vi "Parse NMEA.vi"(8 "error in (no error)":errorcluster, 11 "NMEA Line":string) -> (0 "error out":errorcluster, 3 "NMEA Message out":refnum<class "NMEA Message.lvclass">)   [LabVIEW 2020, in "nmea.lvlib" / "NMEA Message.lvclass"]
uses:
  NMEA Message.lvclass
  NMEA Message.lvclass/NMEA Message.ctl
  <vilib>/Utility/error.llb/Error Cluster From Error Code.vi
  <vilib>/ErrorRing/Error Ring.xnode
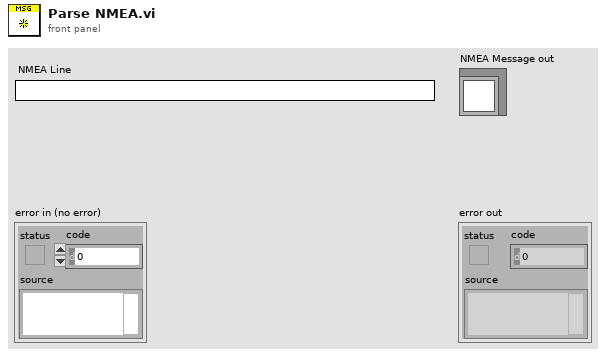
[diagram p1: front panel]
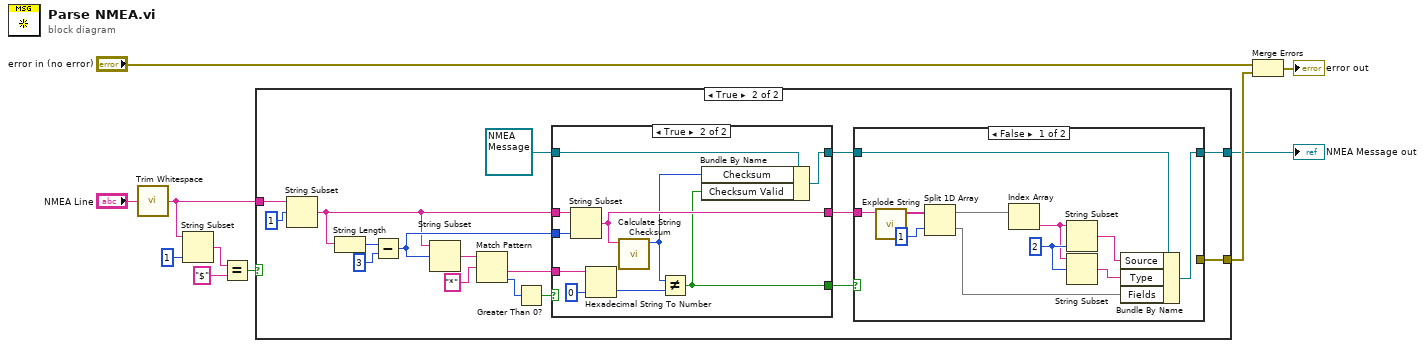
[diagram p0: block diagram]
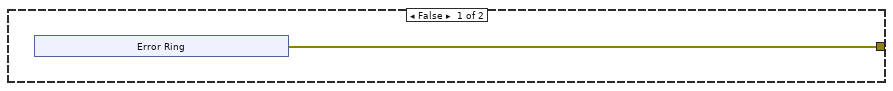
[diagram p2: hidden frame]
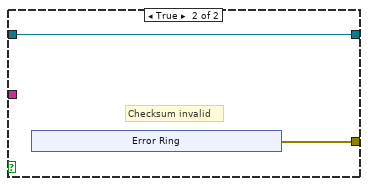
[diagram p4: hidden frame]
diagram:
  n1 = call <vilib>:"Trim Whitespace.vi"("string"="NMEA Line") -> ("trimmed string"=w4:string)  [unwired: 1 in]
  n2 = String Subset(string=w4, length (rest)=1 ("length (rest)")) -> (substring=w8:string)  [unwired: 1 in]
  n3 = Equal?(x=w8, y="$") -> (x = y?=w6:bool)
  n4 = case shown="True" w6 {
    tunnel: w4 -> [_ w15]
    tunnel: [_ w17] -> w1
    tunnel: [w11 w16] -> w2
    frame False {
      n5 = xnode "Error Ring"() -> ("error out"=w11:errorcluster)
    }
    frame True {
      n6 = String Subset(string=w15, offset (0)=1) -> (substring=w14:string)  [unwired: 1 in]
      n7 = String Length(string=w14) -> (length=w29:i32)
      n8 = Subtract(x=w29, y=3) -> (x-y=w27:i32)
      n9 = String Subset(string=w14, offset (0)=w27) -> (substring=w25:string)  [unwired: 1 in]
      n10 = Match Pattern(string=w25, regular expression="*" ("y")) -> (after substring=w21:string, offset past match=w23:i32)  [unwired: 1 in, 2 out]
      n11 = Greater Than 0?(x=w23) -> (x > 0?=w22:bool)
      n12 = case shown="True" w22 {
        tunnel: w14 -> [w31 w41]
        tunnel: w27 -> [_ w40]
        tunnel: [w31 w37] -> w26
        tunnel: w21 -> [_ w39]
        tunnel: [_ w33] -> w20
        tunnel: refnum<class "NMEA Message.lvclass"> refnum ("NMEA Message out") -> [w30 w35]
        tunnel: [w30 w32] -> w18
        frame False {
        }
        frame True {
          n13 = String Subset(string=w41, length (rest)=w40) -> (substring=w37:string)  [unwired: 1 in]
          n14 = Hexadecimal String To Number(string=w39, default (0uL)=u8 0) -> (number=w36:u8)  [unwired: 1 in, 1 out]
          n15 = call "Calculate String Checksum.vi"("String"=w37) -> ("Checksum"=w34:u8)  [unwired: 10 in]
          n16 = Not Equal?(x=w34, y=w36) -> (x != y?=w33:bool)
          n17 = Bundle By Name(cluster=w35, "Checksum"=w34, "Checksum Valid"=w33) -> (w32:refnum<class "NMEA Message.lvclass">)
        }
      }
      n18 = case shown="False" w20 {
        tunnel: w26 -> [w52 _]
        tunnel: w18 -> [w46 w54]
        tunnel: [w42 w54] -> w17
        tunnel: [_ w53] -> w16
        frame False {
          w48 = 2 ("length (rest)")
          n19 = call "Explode String.vi"("String"=w52) -> ("Array"=w51:string[])  [unwired: 10 in]
          n20 = Split 1D Array(array=w51, index=1) -> (first subarray=w49:string[], second subarray=w43:string[])
          n21 = Index Array(array=w49) -> (element=w47:string)  [unwired: 1 in]
          n22 = String Subset(string=w47, length (rest)=w48) -> (substring=w45:string)  [unwired: 1 in]
          n23 = String Subset(string=w47, offset (0)=w48) -> (substring=w44:string)  [unwired: 1 in]
          n24 = Bundle By Name(cluster=w46, "Source"=w45, "Type"=w44, "Fields"=w43) -> (w42:refnum<class "NMEA Message.lvclass">)
        }
        frame True {
          # "Checksum invalid"
          n25 = xnode "Error Ring"() -> ("error out"=w53:errorcluster)
        }
      }
    }
  }
  "NMEA Message out" <- w1
  n26 = Merge Errors("error in (no error)", w2) -> (→"error out":errorcluster)
